vi "NEXT FIELD.vi"(8 "error in (no error)":errorcluster, 9 "Boolean":bool, 10 "MagQ in":refnum<queue>, 11 "Queue in":refnum<queue>) -> (0 "error out":errorcluster, 2 "MagQ out":refnum<queue>, 3 "Queue out":refnum<queue>)   [LabVIEW 2025]
uses:
  Downloads/Magnet Array.ctl
  <instrlib>/SMS LabVIEW Drivers/Source Code/Public/PSU Status.ctl
  <instrlib>/SMS LabVIEW Drivers/Source Code/Cryogenic Ltd SMSXXX.lvlib
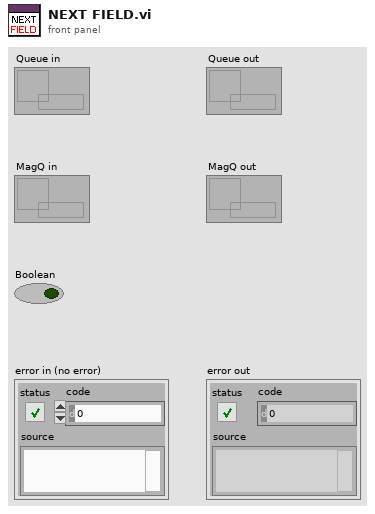
[diagram p1: front panel]
types:
  T1 = enum16{"1. INIT MAG", "2. MAG ON", "3. MAG_STAB", "4. MAG IDLE", "5. PREP NEXT FIELD", "6. APPLY NEXT FIELD", "7. PREP OFF", "8. MAG OFF (Reset)"}
  T2 = typedef "Cryogenic Ltd SMSXXX.lvlib/PSU Status.ctl" = cluster{"Ramp Target":enum16{"ZERO", "MID", "MAX"}, "Pause":bool, "Switch Heater":bool, "Persistent Field":dbl, "Persistent Current":dbl, "Tesla":bool, "Output (T)":dbl, "Output (A)":dbl, "X Trip":enum16{"DISABLED", "ENABLED", "ACTIVE"}, "Ramp Rate (A/s)":dbl, "V Limit (V)":dbl, "Heater Voltage":dbl, "MAX Setpoint (A)":dbl, "MAX Setpoint (T)":dbl, "MID Setpoint (A)":dbl, "MID Setpoint (T)":dbl, "Lock":bool, "Field Constant":dbl, "Remote":bool, "Direction":enum16{"POSITIVE", "NEGATIVE", "OPEN", "UNIPOLAR"}, "Helium Level":u16, "Quench !":bool, "Voltage":dbl, "V Limit !":bool, "Ramping":bool, "At Target":bool, "Trip Field":dbl, "Trip Current":dbl, "Enum":enum16{"1. INIT MAG", "2. MAG ON ", "3. MAG_STAB", "4. MAG IDLE", "5. NEXT FIELD", "6. MAG OFF (Reset)"}}
  T3 = enum16{"SET FIELD", "SWEEP IDLE", "NEXT FIELD", "SWEEP DONE"}
  T4 = typedef "Magnet Array.ctl" = cluster{"Sweep States":enum16{"SET FIELD", "SWEEP IDLE", "NEXT FIELD", "SWEEP DONE"}, "VISA Connection":refnum<visa-resource-name>, "Fields(T)":dbl[]}
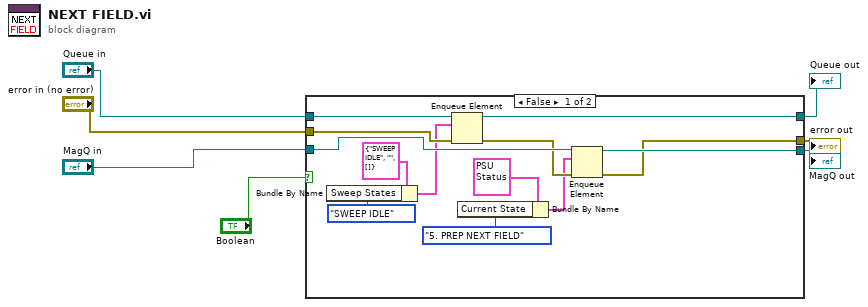
[diagram p0: block diagram]
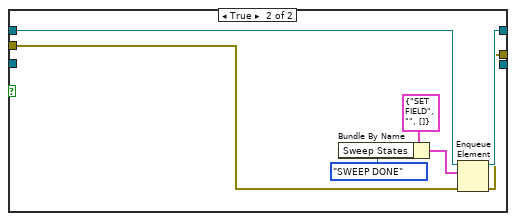
[diagram p2: hidden frame]
diagram:
  n1 = case shown="False" "Boolean" {
    tunnel: "Queue in" -> [w20 w27]
    tunnel: [w19 w26] -> w2
    tunnel: "error in (no error)" -> [w14 w25]
    tunnel: [w12 w24] -> w4
    tunnel: [w18 _] -> w7
    tunnel: "MagQ in" -> [w17 _]
    frame False {
      n2 = Bundle By Name(cluster=T4 {"Sweep States"=enum."SWEEP IDLE", "VISA Connection"="", "Fields(T)"=[]} ("element"), "Sweep States"=T3."SWEEP IDLE") -> (w11:T4)
      n3 = Enqueue Element(queue=w20, element=w11, error in (no error)=w14) -> (queue out=w19:refnum<queue>, error out=w13:errorcluster)  [unwired: 1 in, 1 out]
      n4 = Bundle By Name(cluster=T2 {"Ramp Target"=enum."ZERO", "Pause"=FALSE, "Switch Heater"=FALSE, "Persistent Field"=0.0, "Persistent Current"=0.0, "Tesla"=FALSE, "Output (T)"=0.0, "Output (A)"=0.0, "X Trip"=enum."DISABLED", "Ramp Rate (A/s)"=0.0, "V Limit (V)"=0.0, "Heater Voltage"=0.0, "MAX Setpoint (A)"=0.0, "MAX Setpoint (T)"=0.0, "MID Setpoint (A)"=0.0, "MID Setpoint (T)"=0.0, "Lock"=FALSE, "Field Constant"=0.0, "Remote"=FALSE, "Direction"=enum."POSITIVE", "Helium Level"=0, "Quench !"=FALSE, "Voltage"=0.0, "V Limit !"=FALSE, "Ramping"=FALSE, "At Target"=FALSE, "Trip Field"=0.0, "Trip Current"=0.0, "Enum"=enum."1. INIT MAG"} ("PSU Status In"), "Current State"=T1."5. PREP NEXT FIELD") -> (w9:T2)
      n5 = Enqueue Element(queue=w17, element=w9, error in (no error)=w13) -> (queue out=w18:refnum<queue>, error out=w12:errorcluster)  [unwired: 1 in, 1 out]
    }
    frame True {
      n6 = Bundle By Name(cluster=T4 {"Sweep States"=enum."SET FIELD", "VISA Connection"="", "Fields(T)"=[]} ("element"), "Sweep States"=T3."SWEEP DONE") -> (w21:T4)
      n7 = Enqueue Element(queue=w27, element=w21, error in (no error)=w25) -> (queue out=w26:refnum<queue>, error out=w24:errorcluster)  [unwired: 1 in, 1 out]
    }
  }
  "MagQ out" <- w7
  "error out" <- w4
  "Queue out" <- w2
